vi "Hex String to Byte Array.vi"(11 "Hex String":string) -> (3 "Byte Array":u8[](array[numeric]))   [LabVIEW 2021, in "dotNET Crypto Utility.lvlib"]
doc: "Converts a hex string to a byte array.\n\nWill remove whitespace before converting."
uses:
  dotNET Crypto Utility.lvlib
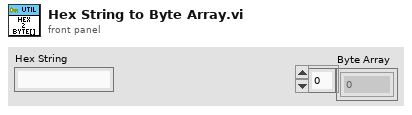
[diagram p1: front panel]
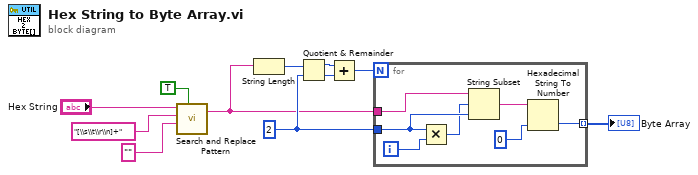
[diagram p0: block diagram]
diagram:
  w7 = i16 2 ("width (-)")
  n1 = call <vilib>:"Search and Replace Pattern.vi"("string"="Hex String", "regular expression (\"\")"="[\\s\\t\\r\\n]+" ("regular expression (\"\")"), "replace string (\"\")"="" ("replace string (\"\")"), "replace all? (F)"=TRUE) -> ("result string"=w3:string)  [unwired: 1 in, 1 out]
  n2 = String Length(string=w3) -> (length=w11:i32)
  n3 = Quotient & Remainder(x=w11, y=w7) -> (x-y*floor(x/y)=w9:i32, floor(x/y)=w10:i32)
  n4 = Add(x=w9, y=w10) -> (x+y=w8:i32)
  n5 = for {
    N: w8 -> [_]
    tunnel: w3 -> [w18]
    tunnel: w7 -> [w16]
    tunnel: [w14] -> w6 mode=indexing
    i -> [w17]
    n6 = Multiply(x=w16, y=w17) -> (x*y=w15:i32)
    n7 = String Subset(string=w18, offset (0)=w15, length (rest)=w16) -> (substring=w12:string)
    n8 = Hexadecimal String To Number(string=w12, default (0uL)=u8 0) -> (number=w14:u8)  [unwired: 1 in, 1 out]
  }
  "Byte Array" <- w6
